vi "Save VI at Path.vi"(5 "Save a Copy (F)":bool, 6 "Without Diagram (F)":bool, 7 "Override Existing? (T)":bool=TRUE, 8 "error in (no error)":errorcluster, 10 "Path":path, 11 "VI in":refnum<vi>) -> (0 "error out":errorcluster, 2 "Path to saved File":path, 3 "VI out":refnum<vi>)   [LabVIEW 2019, in "gRPC Scripting Tools.lvlib"]
uses:
  gRPC Scripting Tools.lvlib
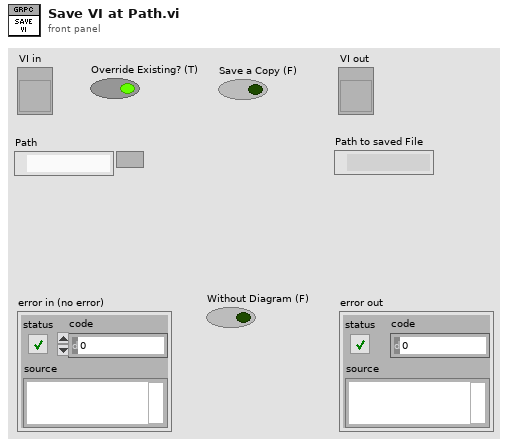
[diagram p1: front panel]
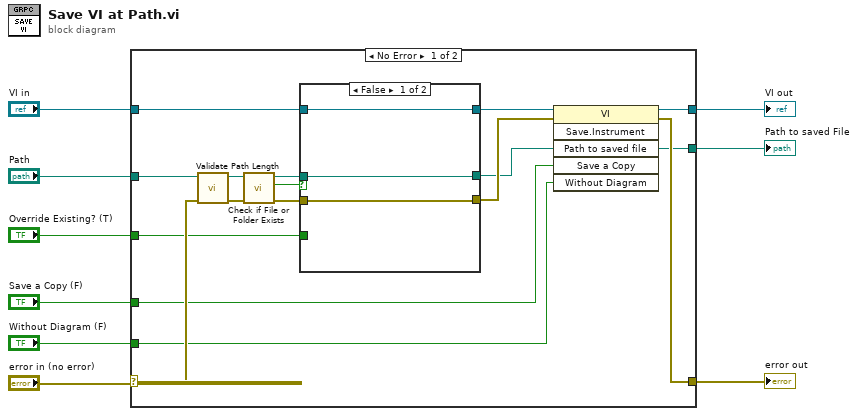
[diagram p0: block diagram]
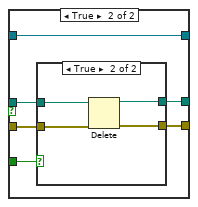
[diagram p2: hidden frame]
diagram:
  n1 = case shown="No Error" "error in (no error)" {
    selector: "error in (no error)" -> [w24 w42]
    tunnel: "Path" -> [w11 w41]
    tunnel: "VI in" -> [w25 w43]
    tunnel: [w14 w42] -> w7
    tunnel: [w19 w43] -> w6
    tunnel: "Save a Copy (F)" -> [w16 _]
    tunnel: "Without Diagram (F)" -> [w15 _]
    tunnel: "Override Existing? (T)" -> [w18 _]
    tunnel: [w13 w41] -> w1
    frame No Error {
      n2 = call "Validate Path Length.vi"("error in (no error)"=w24, "Path in"=w11) -> ("error out"=w12:errorcluster, "Path out"=w10:path)  [unwired: 8 in]
      n3 = call <vilib>:"Check if File or Folder Exists.vi"("error in (no error)"=w12, "path"=w10) -> ("error out"=w21:errorcluster, "file or folder exists?"=w22:bool, "dup path"=w23:path)  [unwired: 7 in]
      n4 = case shown="False" w22 {
        tunnel: w25 -> [w28 w34]
        tunnel: [w28 w34] -> w20
        tunnel: w23 -> [w26 w33]
        tunnel: w21 -> [w27 w32]
        tunnel: [w26 w31] -> w13
        tunnel: [w27 w30] -> w17
        tunnel: w18 -> [_ w29]
        frame False {
        }
        frame True {
          n5 = case shown="True" w29 {
            tunnel: w33 -> [w36 w40]
            tunnel: w32 -> [w35 w39]
            tunnel: [w36 w38] -> w31
            tunnel: [w35 w37] -> w30
            frame False {
            }
            frame True {
              n6 = Delete(path (use dialog)=w40, error in=w39) -> (deleted path=w38:path, error out=w37:errorcluster)  [unwired: 3 in, 1 out]
            }
          }
        }
      }
      n7 = invoke class="VI" method="Save.Instrument"(reference=w20, error in=w17, "Path to saved file"=w13, "Save a Copy"=w16, "Without Diagram"=w15) -> (reference out=w19:refnum<vi>, error out=w14:errorcluster)  [unwired: 1 in, 4 out]
    }
    frame Error {
    }
  }
  "error out" <- w7
  "VI out" <- w6
  "Path to saved File" <- w1
